vi "Concept of LOG_host.vi"() -> ()   [LabVIEW 2011]
uses:
  <vilib>/rvi/FXPMathLib/FxpInterpret/XNode/nifxpmath_Interpret.xnode
panel:
  out "log{Mantissa}":fxp<+/-,18,8> format="%.13g"
  out "log2 (+/-,25,3)":fxp<+/-,25,3> format="%.23g"
  out "Truncated Address":u16
  out "Mantissa (M)":u32
  out "Exponent (-N)":i8
  out "Error (DBL and FXP)":dbl
  out "LUT calculation":fxp<+/-,33,11> format="%.26g"
  out "LUT":fxp<+/-,18,8>[](array[numeric]) format="%.13g"
  out "dB (DBL, log10)":dbl
  in  "Input Number (1.32)":fxp<+,32,1>
  # "Output"
  # "Test Cases for Magnitude\n2.32831E-10\n1\n0\n0.567893\n0.06967"
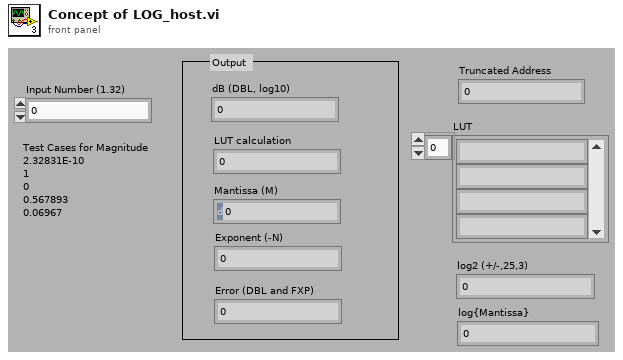
[diagram p1: front panel]
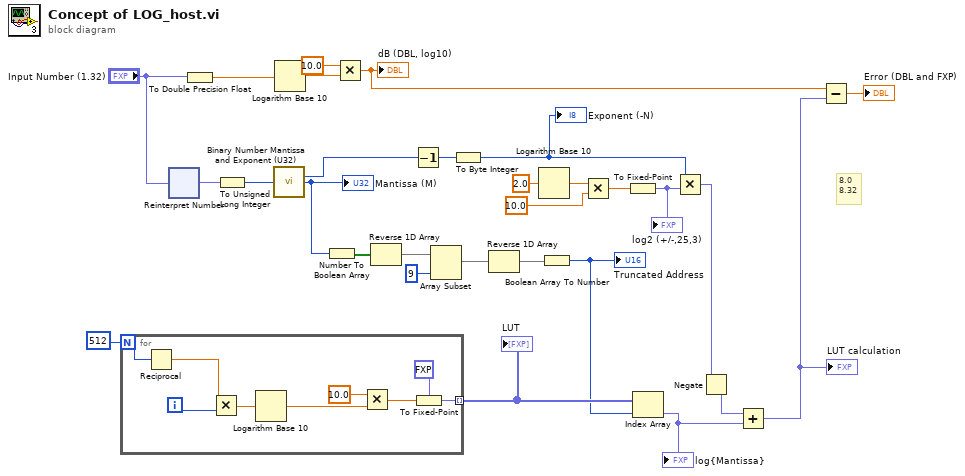
[diagram p0: block diagram]
diagram:
  # "8.0\n8.32"
  n1 = for {
    N: 512 -> [w38]
    tunnel: [w33] -> w25 mode=indexing
    i -> [w36]
    n2 = Reciprocal(x=w38) -> (1/x=w37:dbl)
    n3 = Multiply(x=w37, y=w36) -> (x*y=w32:dbl)
    n4 = Logarithm Base 10(1:w32) -> (0:w34:dbl)
    n5 = Multiply(x=10.0, y=w34) -> (x*y=w30:dbl)
    n6 = To Fixed-Point(fixed-point type=fxp<+/-,18,8> 0.0, number=w30) -> (fixed-point=w33:fxp<+/-,18,8>)
  }
  "LUT" <- w25
  n7 = xnode "Reinterpret Number"("x"="Input Number (1.32)") -> ("y"=w22:fxp<+,32,32>)
  n8 = To Double Precision Float(number="Input Number (1.32)") -> (double precision float=w29:dbl)
  n9 = To Unsigned Long Integer(number=w22) -> (unsigned 32bit integer=w21:u32)
  n10 = call <userlib>:"Binary Number Mantissa and Exponent (U32).vi"("Binary Number"=w21) -> ("Exponent (-N)"=w11:i8, "Mantissa (M)"=w12:u32)  [unwired: 12 in, 1 out]
  "Mantissa (M)" <- w12
  n11 = Logarithm Base 10(1:w29) -> (0:w28:dbl)
  n12 = Number To Boolean Array(number=w12) -> (Boolean array=w19:bool[])
  n13 = Multiply(x=10.0, y=w28) -> (x*y=w24:dbl)
  "dB (DBL, log10)" <- w24
  n14 = Reverse 1D Array(array=w19) -> (reversed array=w18:bool[])
  n15 = Decrement(x=w11) -> (x-1=w3:i8)
  n16 = Array Subset(array=w18, length=9) -> (w16:bool[])  [unwired: 1 in]
  n17 = To Byte Integer(number=w3) -> (8bit integer=w2:i8)
  "Exponent (-N)" <- w2
  n18 = Reverse 1D Array(array=w16) -> (reversed array=w15:bool[])
  n19 = Logarithm Base 10(1:2.0 ("x")) -> (0:w8:dbl)
  n20 = Boolean Array To Number(Boolean array=w15) -> (number=w17:u16)
  "Truncated Address" <- w17
  n21 = Multiply(x=w8, y=10.0) -> (x*y=w6:dbl)
  n22 = To Fixed-Point(number=w6) -> (fixed-point=w5:fxp<+/-,25,3>)  [unwired: 1 in]
  "log2 (+/-,25,3)" <- w5
  n23 = Index Array(array=w25, index=w17) -> (element=w14:fxp<+/-,18,8>)
  "log{Mantissa}" <- w14
  n24 = Multiply(x=w2, y=w5) -> (x*y=w4:fxp<+/-,33,11>)
  n25 = Negate(x=w4) -> (-x=w1:fxp<+/-,32,10>)
  n26 = Add(x=w1, y=w14) -> (x+y=w13:fxp<+/-,33,11>)
  "LUT calculation" <- w13
  n27 = Subtract(x=w24, y=w13) -> (x-y=→"Error (DBL and FXP)":dbl)
